vi "AB_Engine_Get_LV_IconNameMac.vi"(8 "error in (no error)":errorcluster, 11 "use version independent app":bool) -> (0 "error out":errorcluster, 3 "icon file name":string)   [LabVIEW 2020]
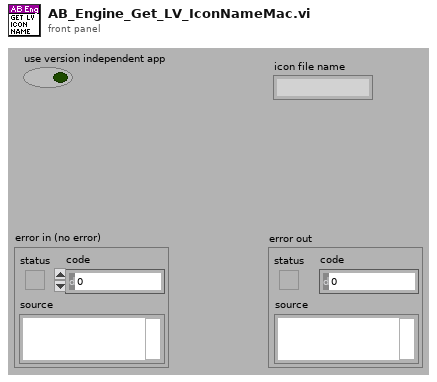
[diagram p1: front panel]
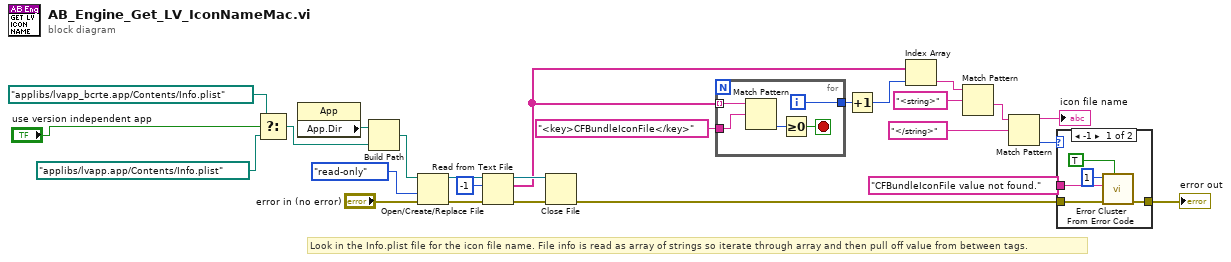
[diagram p0: block diagram]
diagram:
  # "Look in the Info.plist file for the icon file name. File info is read as array of strings so iterate through array and then pull off value from between tags."
  n1 = Select(t=path "applibs/lvapp_bcrte.app/Contents/Info.plist", s="use version independent app", f=path "applibs/lvapp.app/Contents/Info.plist") -> (s? t:f=w1:path)
  n2 = property class="App"() -> ("App.Dir"=w11:path)  [unwired: 2 in, 2 out]
  n3 = Build Path(base path=w11, name or relative path=w1) -> (appended path=w10:path)
  n4 = Open/Create/Replace File(file path (use dialog)=w10, error in="error in (no error)", access (0:read/write)=enum16{"read/write", "read-only", "write-only"}."read-only") -> (refnum out=w26:refnum<file>, error out=w23:errorcluster)  [unwired: 3 in, 1 out]
  n5 = Read from Text File(file (use dialog)=w26, count=-1, error in=w23) -> (refnum out=w24:refnum<file>, text=w19:string[], error out=w22:errorcluster)  [unwired: 1 in, 1 out]
  n6 = Close File(refnum=w24, error in=w22) -> (error out=w8:errorcluster)  [unwired: 1 out]
  n7 = for {
    tunnel: w19 -> [w31] mode=indexing
    tunnel: "<key>CFBundleIconFile</key>" -> [w30]
    tunnel: [w27] -> w18
    i -> [w27]
    stop <- w28 stop-if-true
    n8 = Match Pattern(string=w31, regular expression=w30) -> (offset past match=w29:i32)  [unwired: 1 in, 3 out]
    n9 = Greater Or Equal To 0?(x=w29) -> (x >= 0?=w28:bool)
  }
  n10 = Increment(x=w18) -> (x+1=w17:i32)
  n11 = Index Array(array=w19, index=w17) -> (element=w16:string)
  n12 = Match Pattern(string=w16, regular expression="<string>") -> (after substring=w13:string)  [unwired: 1 in, 3 out]
  n13 = Match Pattern(string=w13, regular expression="</string>") -> (before substring=→"icon file name":string, offset past match=w7:i32)  [unwired: 1 in, 2 out]
  n14 = case shown="-1" w7 {
    tunnel: w8 -> [w36 w37]
    tunnel: [w35 w37] -> w6
    tunnel: "CFBundleIconFile value not found." -> [w34 _]
    frame -1 {
      n15 = call <vilib>:"Error Cluster From Error Code.vi"("show call chain? (False)"=TRUE, "error in (no error)"=w36, "error message (\"\")"=w34, "error code (0)"=1) -> ("error out"=w35:errorcluster)  [unwired: 5 in]
    }
    frame Default {
    }
  }
  "error out" <- w6
